vi "Shut_down_EnFlo_Tunnel.vi"(3 "Mode":T5, 5 "Traverse line In":T2 {"Row Duration (mins)" format="%#.1f"; "Row No" min=0; "Trace Gas Concentration (%)" min=0.0 format="%#.2f"; "Emission Rate (l/min)" format="%#.2f"; "Tunnel Speed" format="%#.2f"; "Start X" format="%#.2f"; "Start Y" format="%#.2f"; "Start Z" format="%#.2f"; "End X" format="%#.2f"; "End Y" format="%#.2f"; "End Z" format="%#.2f"; "Averaging time (min)" min=0.0 format="%#.2f"}) -> (0 "Error Message":string, 1 "Status":T1, 2 "Traverse line Out":T2 {"Row Duration (mins)" format="%#.1f"; "Row No" min=0; "Trace Gas Concentration (%)" min=0.0 format="%#.2f"; "Emission Rate (l/min)" format="%#.2f"; "Tunnel Speed" format="%#.2f"; "Start X" format="%#.2f"; "Start Y" format="%#.2f"; "Start Z" format="%#.2f"; "End X" format="%#.2f"; "End Y" format="%#.2f"; "End Z" format="%#.2f"; "Averaging time (min)" min=0.0 format="%#.2f"})   [LabVIEW 2013]
uses:
  Gen Trav/Traverse_cluster.ctl
  Gen Trav/Spacing.ctl
  Controls/Multi_run_mode.ctl
  Controls/User_Specific_mode.ctl
  Gen Trav/Multi_Run_Status.ctl
  ADAM Client/Sub VIs/ADAM Controls/Update_scan_value.ctl
  ADAM Client/Sub VIs/ADAM Controls/Tunnel_speed_mode.ctl
panel:
  # "X           Y            Z"
  # "Start"
  # "End"
  # "X           Y            Z"
  # "Start"
  # "End"
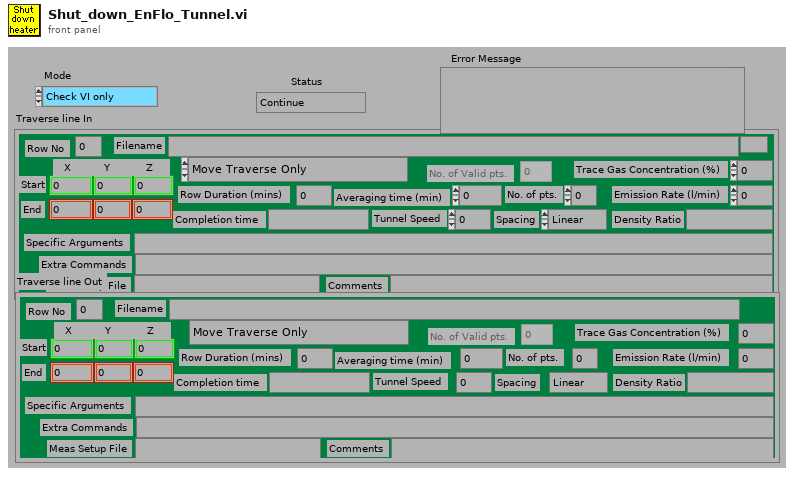
[diagram p1: front panel]
types:
  T1 = typedef "Multi_Run_Status.ctl" = enum16{"Continue", "Jump to Next Point", "Jump to Next Row", "Jump To Fall Back", "Terminate Run"}
  T2 = typedef "Traverse_cluster.ctl" = cluster{"Start X":dbl, "Start Y":dbl, "Start Z":dbl, "End X":dbl, "End Y":dbl, "End Z":dbl, "No. of pts.":i32, "Spacing":T3, "Filename":path, "Tunnel Speed":dbl, "Averaging time (min)":dbl, "Extra Commands":string, "Specific Arguments":string, "Emission Rate (l/min)":dbl, "Trace Gas Concentration (%)":dbl, "Density Ratio":string, "Comments":string, "Row No":i32, "Row Type Selector":T4, "Completion time":string, "Row Duration (mins)":dbl, "No. of Valid pts.":i32, "Meas Setup File":string}
  T3 = typedef "Spacing.ctl" = enum16{"Linear", "Log", "Gauss", "Specified", "N/A"}
  T4 = typedef "Multi_run_mode.ctl" = enum16{"Move Traverse Only", "Set Tunnel Speed Only", "Set Source Only", "Set Measurement Conditions", "Single Measurement", "Vertical Profile", "Lateral Profile", "Longitudinal Profile", "Explore Volume", "Multi-Axis Profile", "Auto Calibrate", "Meas Fast FID Bkgnd", "Check Beam Power", "Scanning Valve Measurement", "Run VI Named:", "Set ADAM Ch", "Wait (minutes)", "Send Message", "Synchronize With:", "Fall Back to this Row", "Turn Off Row Repeating", "Blank Row", "Traverse 3D Volume"}
  T5 = typedef "User_Specific_mode.ctl" = enum16{"Check VI only", "Run VI"}
  T6 = typedef "Update_scan_value.ctl" = cluster{"Channel Name":string, "New Value":dbl}
  T7 = typedef "Tunnel_speed_mode.ctl" = enum16{"Set Speed", "Set Speed then wait", "Is tunnel speed allowable?"}
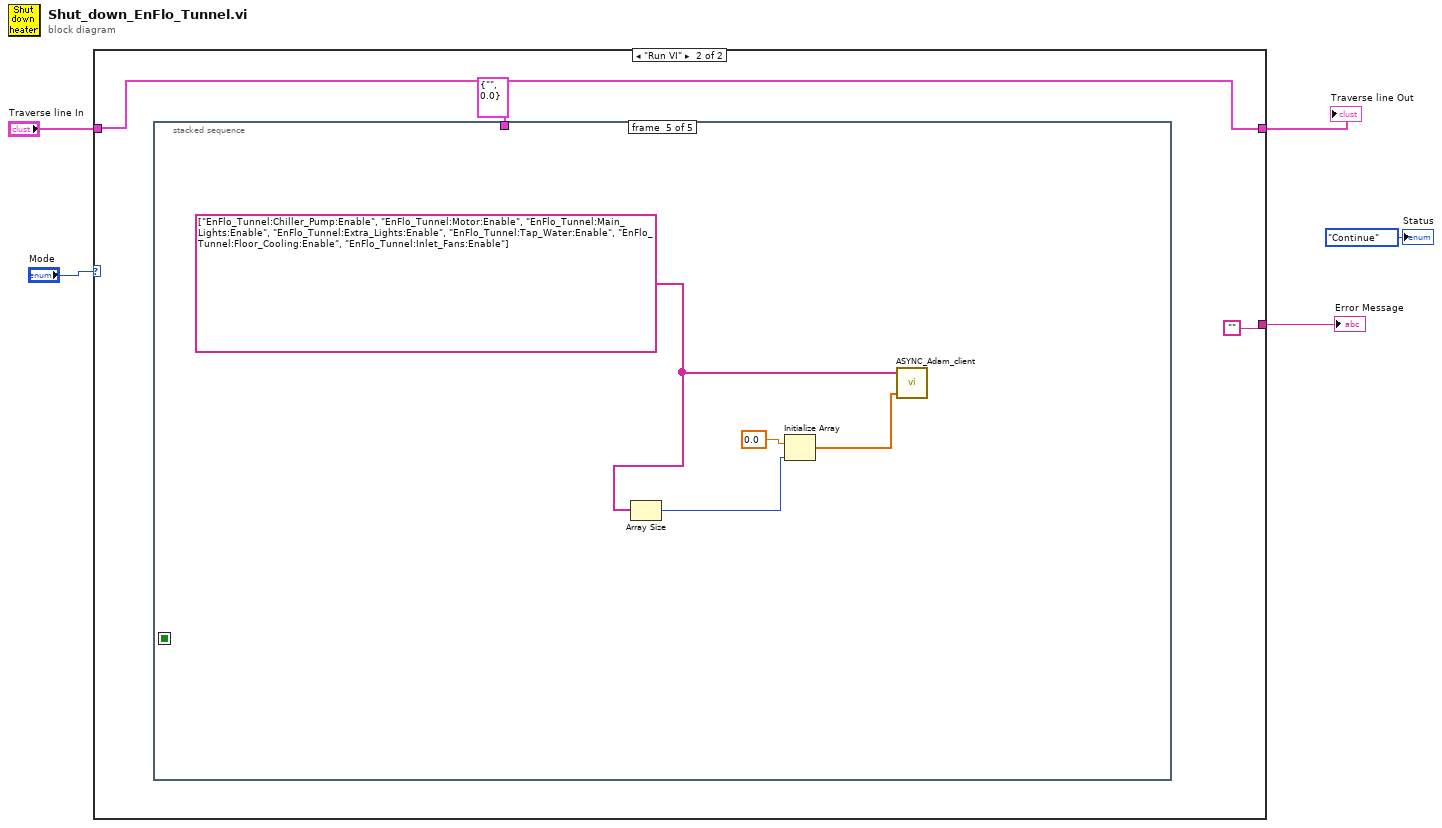
[diagram p0: block diagram]
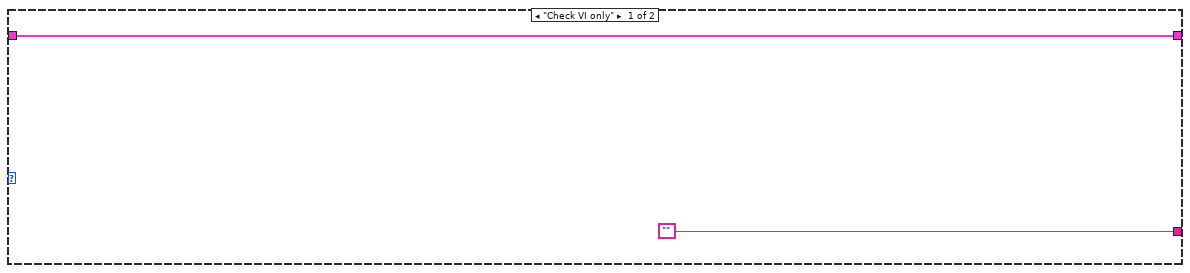
[diagram p2: hidden frame]
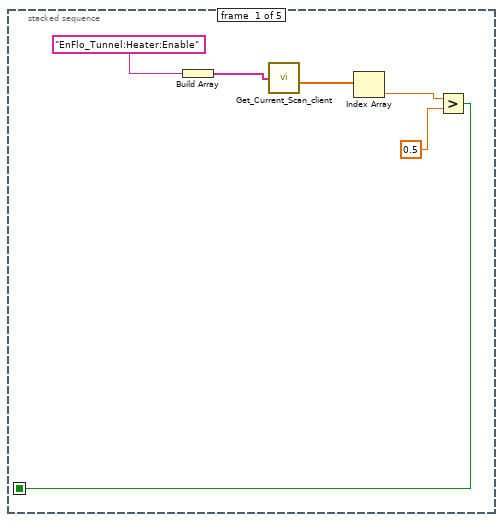
[diagram p3: hidden frame]
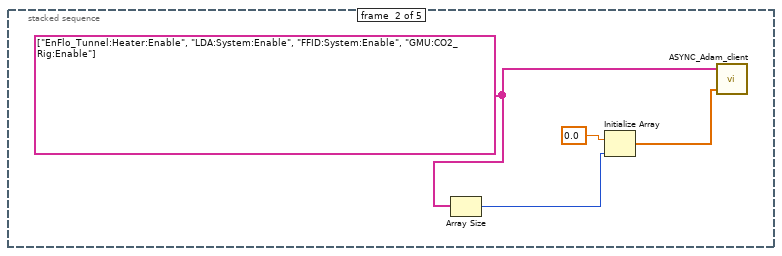
[diagram p4: hidden frame]
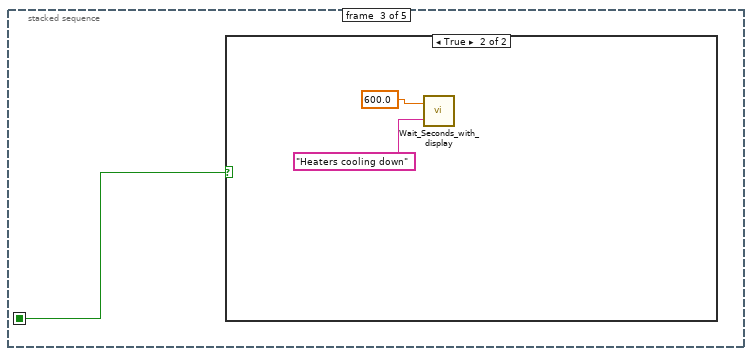
[diagram p5: hidden frame]
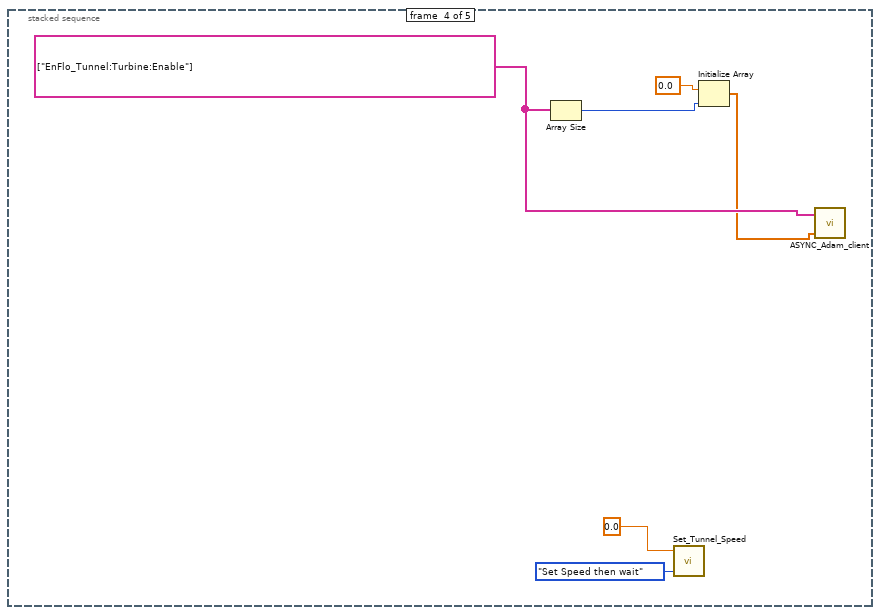
[diagram p7: hidden frame]
diagram:
  n1 = case shown="\"Run VI\"" "Mode" {
    tunnel: "Traverse line In" -> [w7 w9]
    tunnel: [w7 w9] -> w3
    tunnel: ["" ""] -> w2
    frame "Check VI only" {
    }
    frame "Run VI" {
      n2 = stacked-sequence {
        seq-local: [w11 _ _ _ _] -> [_ _ w21 _ _]
        tunnel: T6 {"Channel Name"="", "New Value"=0.0} ("Update Scan Value Cluster") -> [_ _ _ _ _]
        frame #0 {
          n3 = Build Array("EnFlo_Tunnel:Heater:Enable") -> (w15:string[])
          n4 = call "Get_Current_Scan_client.vi"("ADAM Ch Names"=w15) -> ("Numerical Values"=w14:dbl[])  [unwired: 1 in, 2 out]
          n5 = Index Array(array=w14) -> (element=w13:dbl)  [unwired: 1 in]
          n6 = Greater?(x=w13, y=0.5) -> (0:w11:bool)
        }
        frame #1 {
          w20 = string[] ["EnFlo_Tunnel:Heater:Enable", "LDA:System:Enable", "FFID:System:Enable", "GMU:CO2_Rig:Enable"] ("appended array")
          n7 = Array Size(array=w20) -> (size(s)=w19:i32)
          n8 = Initialize Array(0.0 ("Input Element"), w19) -> (w18:dbl[])
          n9 = call "ASYNC_Adam_client.vi"("Values"=w18, "Channel Names"=w20) -> ()  [unwired: 1 in, 2 out]
        }
        frame #2 {
          n10 = case shown="True" w21 {
            frame False {
            }
            frame True {
              n11 = call "Wait_Seconds_with_display.vi"("Message"="Heaters cooling down", "Seconds to wait"=600.0) -> ()  [unwired: 2 out]
            }
          }
        }
        frame #3 {
          w25 = string[] ["EnFlo_Tunnel:Turbine:Enable"] ("appended array")
          n12 = Array Size(array=w25) -> (size(s)=w27:i32)
          n13 = call "Set_Tunnel_Speed.vi"("Mode"=Tunnel_speed_mode."Set Speed then wait", "Tunnel Velocity m/s"=0.0) -> ()  [unwired: 3 in, 1 out]
          n14 = Initialize Array(0.0 ("Input Element"), w27) -> (w24:dbl[])
          n15 = call "ASYNC_Adam_client.vi"("Values"=w24, "Channel Names"=w25) -> ()  [unwired: 1 in, 2 out]
        }
        frame #4 {
          w33 = string[] ["EnFlo_Tunnel:Chiller_Pump:Enable", "EnFlo_Tunnel:Motor:Enable", "EnFlo_Tunnel:Main_Lights:Enable", "EnFlo_Tunnel:Extra_Lights:Enable", "EnFlo_Tunnel:Tap_Water:Enable", "EnFlo_Tunnel:Floor_Cooling:Enable", "EnFlo_Tunnel:Inlet_Fans:Enable"] ("appended array")
          n16 = Array Size(array=w33) -> (size(s)=w32:i32)
          n17 = Initialize Array(0.0 ("Input Element"), w32) -> (w31:dbl[])
          n18 = call "ASYNC_Adam_client.vi"("Values"=w31, "Channel Names"=w33) -> ()  [unwired: 1 in, 2 out]
        }
      }
    }
  }
  "Traverse line Out" <- w3
  "Error Message" <- w2
  "Status" <- Multi_Run_Status."Continue" ("Status")
